vi "平均值波形图表显示.vi"() -> ()   [LabVIEW 2012]
uses:
  <vilib>/Analysis/baseanly.llb/Mean (DBL).vi
  <vilib>/Analysis/NI_AALBase.lvlib
panel:
  in  "stop":bool
  out "随机数波形图表":dbl(graph)
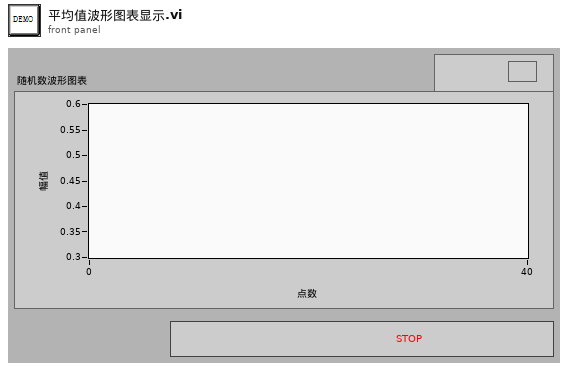
[diagram p1: front panel]
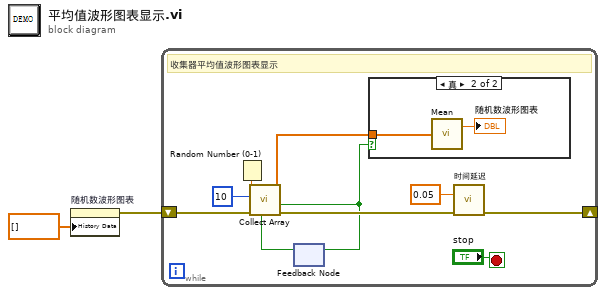
[diagram p0: block diagram]
diagram:
  n1 = property on="随机数波形图表" class="WFChart (严格)"("History Data"=dbl[] [] ("历史数据")) -> (error out=w2:errorcluster)  [unwired: 2 in, 1 out]
  n2 = while {
    shift-right: [w11] -> _
    shift-left: w2 -> [w7]
    stop <- "stop" stop-if-true
    # "收集器平均值波形图表显示"
    n3 = Random Number (0-1)() -> (number: 0 to 1=w9:dbl)
    n4 = feedback #1() -> (w5:bool)  [unwired: 1 in]
    n5 = call-poly "Collect Array.vi"("reset"=w5, "error in"=w7, "array size"=u32 10, "input"=w9) -> ("error out"=w6:errorcluster, "full"=w4:bool, "collected data"=w3:dbl[])  [unwired: 4 in, 1 out]
    n6 = feedback-in #1(w4) -> ()
    n7 = case shown="真" w4 {
      tunnel: w3 -> [_ w14]
      frame False {
      }
      frame True {
        n8 = call-poly <vilib>:"Mean.vi"("X"=w14) -> ("mean"=→"随机数波形图表":dbl)  [unwired: 1 out]
      }
    }
    n9 = call "时间延迟"("error in (no error)"=w6, "Delay Time (s)"=0.05) -> ("error out"=w11:errorcluster)  [unwired: 9 in]
  }
